vi "Filter Control Drag Starting Event.vi"(8 "error in (no error)":errorcluster, 10 "ControlDragStartingMsg":refnum<class "ControlDragStartingMsg.lvclass">, 11 "IEventFilter in":refnum<class "IEventFilter.lvclass">) -> (0 "error out":errorcluster, 1 "Discard?":bool, 2 "Filtered Event Data":T1, 3 "IEventFilter out":refnum<class "IEventFilter.lvclass">, 5 "Data Filtered?":bool)   [LabVIEW 2015, in "ActorEvents.lvlib" / "IEventFilter.lvclass"]
uses:
  IEventFilter.lvclass
  IEventAggregator Messages/ControlDragStartingMsg/ControlDragStartingMsg.lvclass
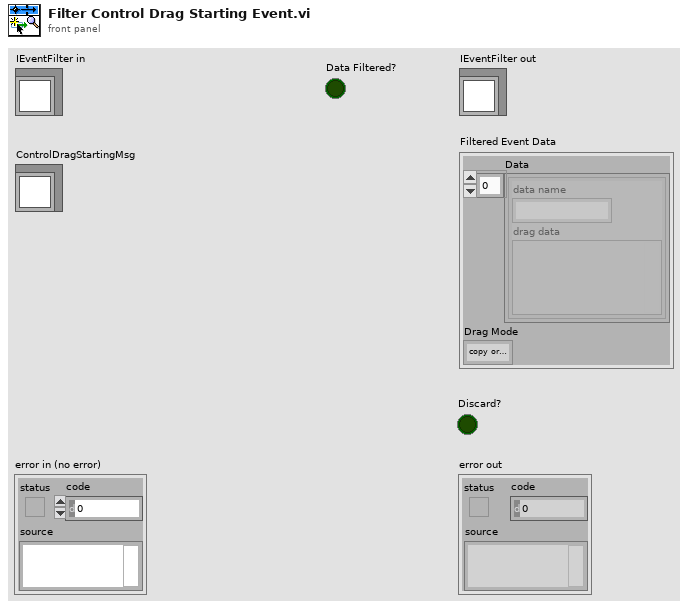
[diagram p1: front panel]
types:
  T1 = cluster{"Data":cluster{"data name":string, "drag data":variant}[], "Drag Mode":enum32{"copy or move", "copy only", "move only"}}
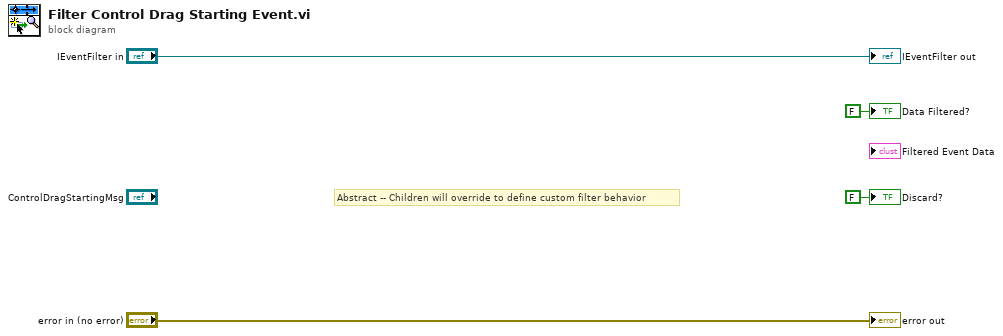
[diagram p0: block diagram]
diagram:
  # "Abstract -- Children will override to define custom filter behavior"
  "error out" <- "error in (no error)"
  "IEventFilter out" <- "IEventFilter in"
  "Discard?" <- FALSE ("Discard?")
  "Data Filtered?" <- FALSE ("Data Filtered?")
